vi "Process.vi"(8 "error in":errorcluster, 11 "instrument.PPMS2":refnum<class "instrument.PPMS2.lvclass">) -> (0 "error out":errorcluster, 3 "instrument.PPMS2 out":refnum<class "instrument.PPMS2.lvclass">)   [LabVIEW 2016, in "instrument.PPMS2.lvclass"]
doc: "---------------------------------------------------------------\nJKI State Machine Objects™\nhttp://jki.net/state-machine-objects/\nCopyright (C) 2005-2015, JKI <info@jki.net>\nALL RIGHTS RESERVED"
uses:
  instrument.PPMS2.lvclass
  C:/Program Files (x86)/National Instruments/LabVIEW 2016/vi.lib/JKI/JKI SMO/SMO/SMO.lvclass
  <vilib>/JKI/JKI SMO/SMO/Typedefs/Parent Call--Enum.ctl
  PPMS Global.vi
  C:/user/patrick/hg/levylab_inst_ppms2/lvsrc/QDInstrument_LabView/QDInstrument.dll
  QDInstrument_LabView/QDInstrument.dll
  <userlib>/LevyLab/Levylab Instruments DELETE ME SOMETIME/Instrument.lvclass
  <vilib>/JKI/JKI SMO/SMO/SMO.lvclass
panel:
  in  "Refresh Rate (Hz)":dbl=13.0
  out "Field Status":i32(ring)=1 items=["MagnetUnknown"=0, "StablePersistent"=1, "WarmingSwitch"=2, "CoolingSwitch"=3, "StableDriven"=4, "Iterating"=5, "Charging"=6, "Discharging"=7, "CurrentError"=8, "MagnetFailure"=15]
  in  "STOP":bool
  in  "Temp Approach":enum16{"FastSettle", "NoOvershoot"}(ring)
  in  "Low Helium Level Notify?":bool
  in  "Helium Notification Level":dbl=1.0
  out "Helium Level":dbl=86.7
  out "Position":dbl=90.002
  out "Field (Oe)":dbl=-0.00643419474363327 format="%_3g"
  out "Temperature(K)":dbl=305.0156 format="%#_5g"
  out "Temperature Status":T1(ring)=enum."Stable"
  in  "IP Address":string="130.49.180.72"
  # "PPMS2 Monitor Control"
  # "For instructions on how to use the JKI State Machine Objects, examples and video tutorials, visit:\nhttp://jki.net/state-machine-objects/\n\nJKI State Machine Objects™\nhttp://jki.net/state-machine-objects/\nCopyright (C) 2005-2015, JKI <info@jki.net>\nALL RIGHTS RESERVED"
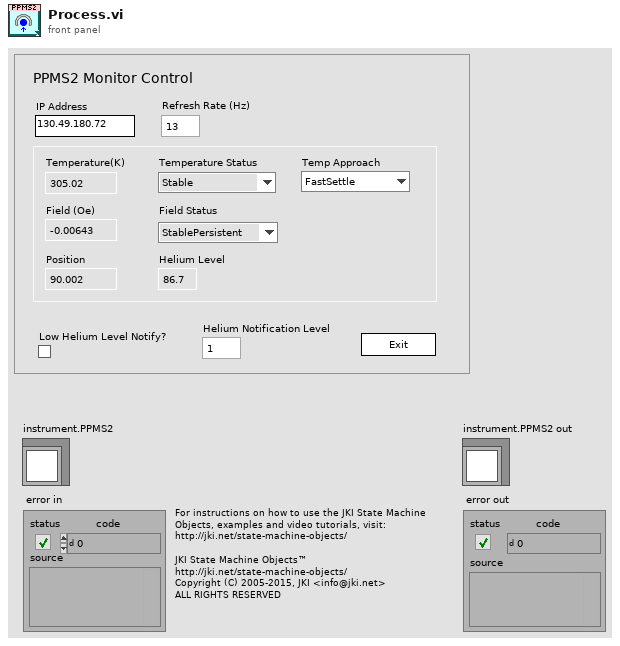
[diagram p1: front panel]
types:
  T1 = enum16{"TemperatureUnknown", "Stable", "Tracking", "Near", "Chasing", "Filling", "Standby", "Disabled", "ImpedanceNotFunction", "TempFailure"}
  T2 = typedef "SMO.lvclass/Parent Call--Enum.ctl" = enum16{"Allows parent to run", "Does not request parent to run"}
  T3 = enum32{"invalid app kind", "Development System", "Run Time System", "Student Edition", "Embedded LabVIEW", "Evaluation", "Custom"}
  T4 = enum32{"Invalid", "Standard", "Closed", "Hidden", "Minimized", "Maximized"}
  T5 = enum32{"Bad", "Idle", "Run top level", "Running"}
  T6 = enum16{"0", "1", "2", "3", "4", "5", "6", "7", "8", "9", "10", "11", "12", "13", "14"}
  T7 = cluster{"Core":cluster{"Current VI Reference":refnum<vi>, "Close Panel on Exit?":bool, "error":errorcluster}, "Self Reference":refnum<class "instrument.PPMS2.lvclass">, "to":i32, "Instrument Ref":refnum<k24>}
  T8 = cluster{"Current VI Reference":refnum<vi>, "Close Panel on Exit?":bool, "error":errorcluster}
  T9 = typedef "SMO.lvclass/Protected Events.ctl" = cluster{"StopProcesses":refnum<user-event>, "AbortProcesses":refnum<user-event>, "Config Changed":refnum<user-event>, "Dependency":refnum<user-event>}
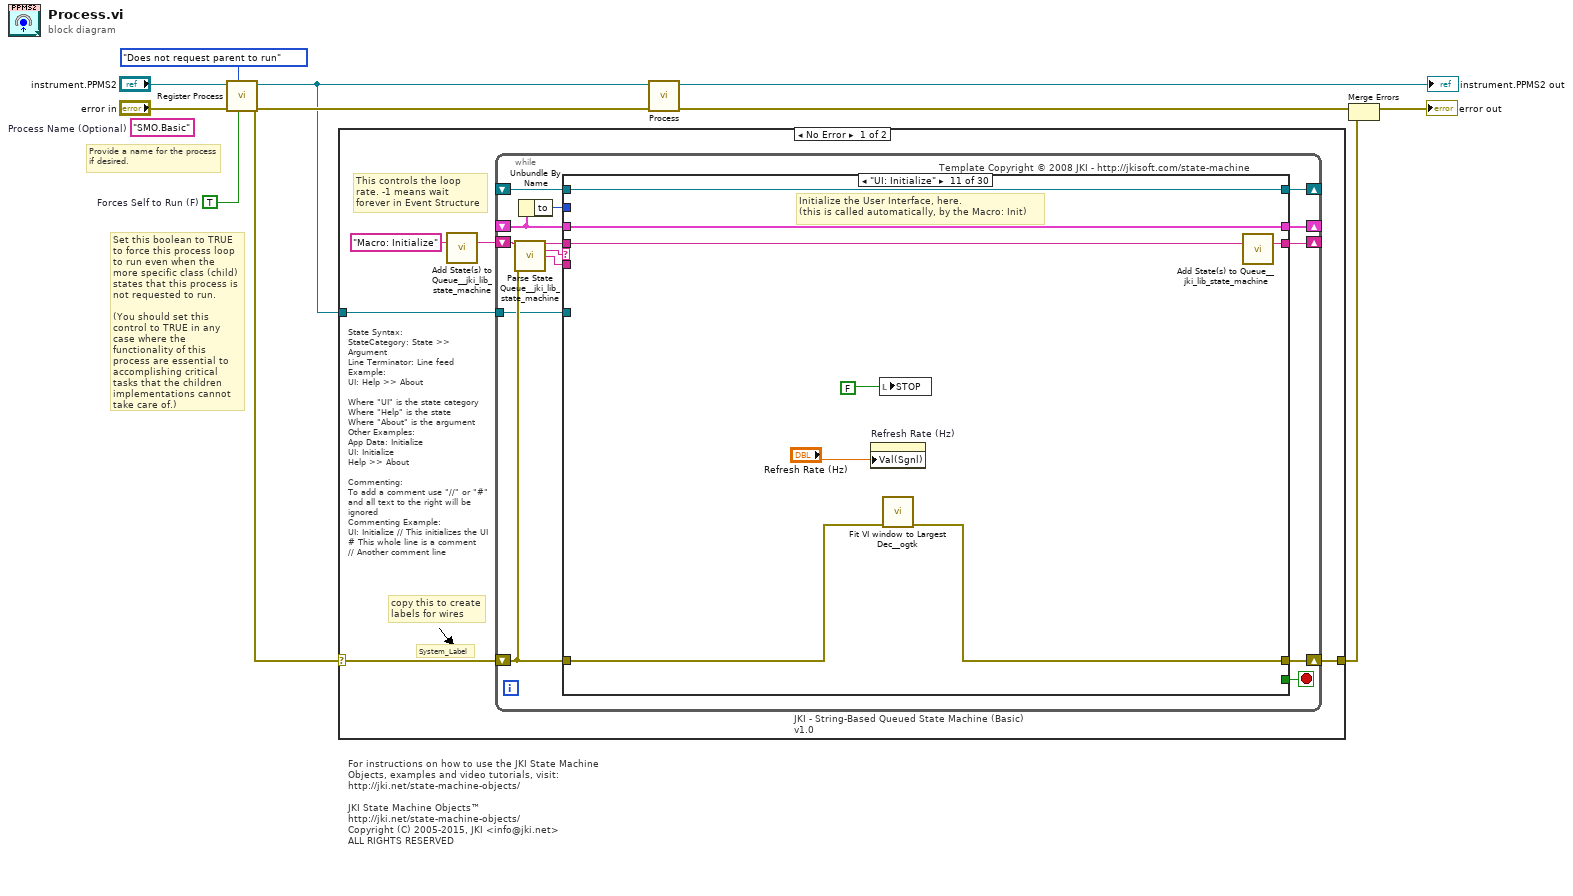
[diagram p0: block diagram]
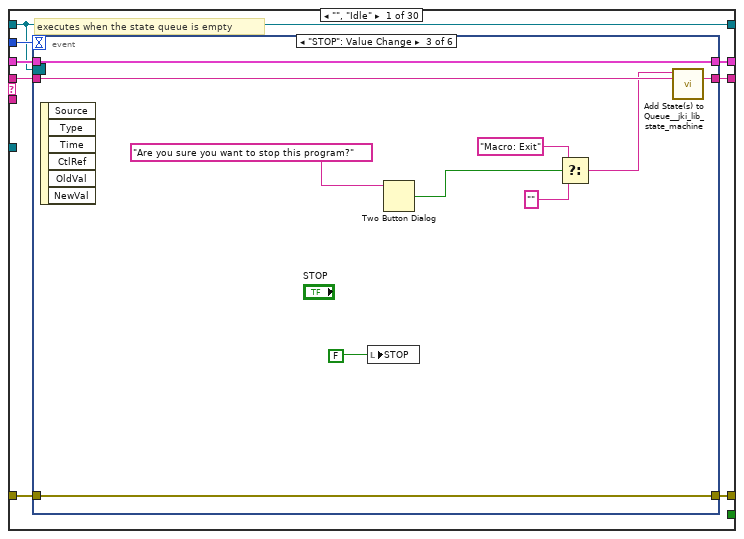
[diagram p2: hidden frame]
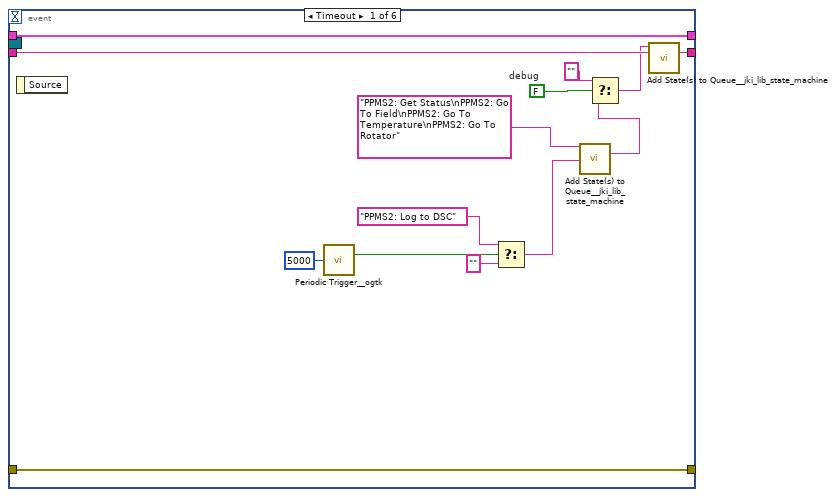
[diagram p3: hidden frame]
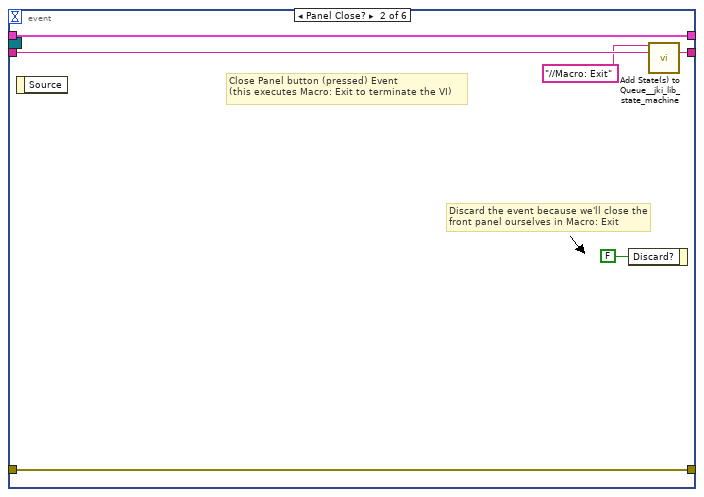
[diagram p4: hidden frame]
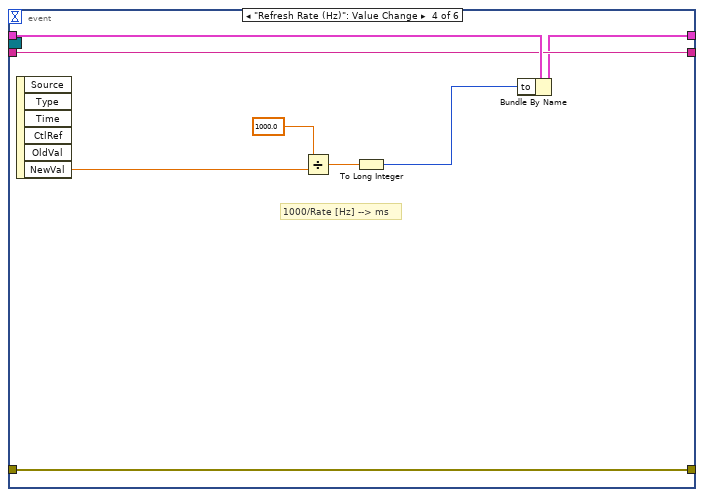
[diagram p5: hidden frame]
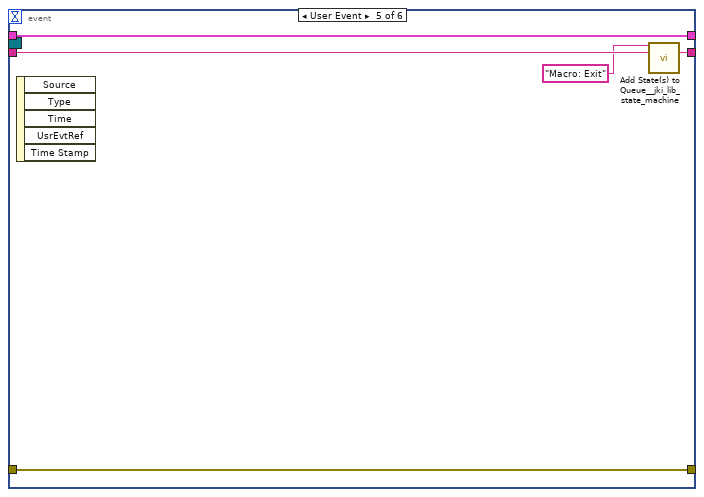
[diagram p6: hidden frame]
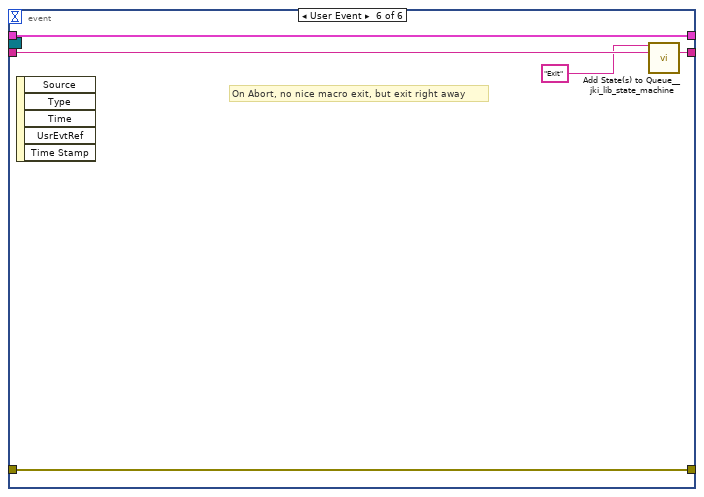
[diagram p7: hidden frame]
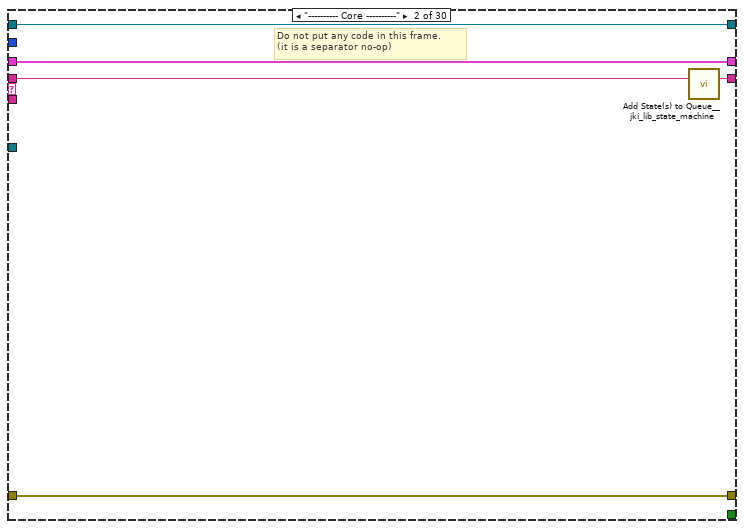
[diagram p8: hidden frame]
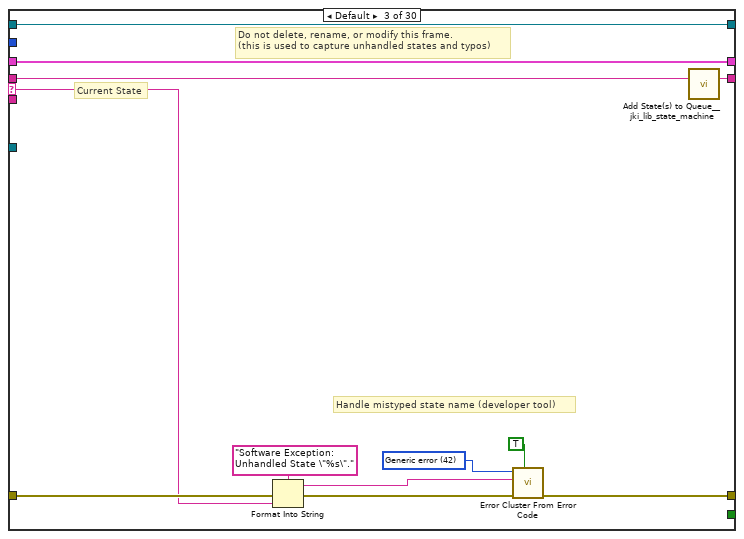
[diagram p9: hidden frame]
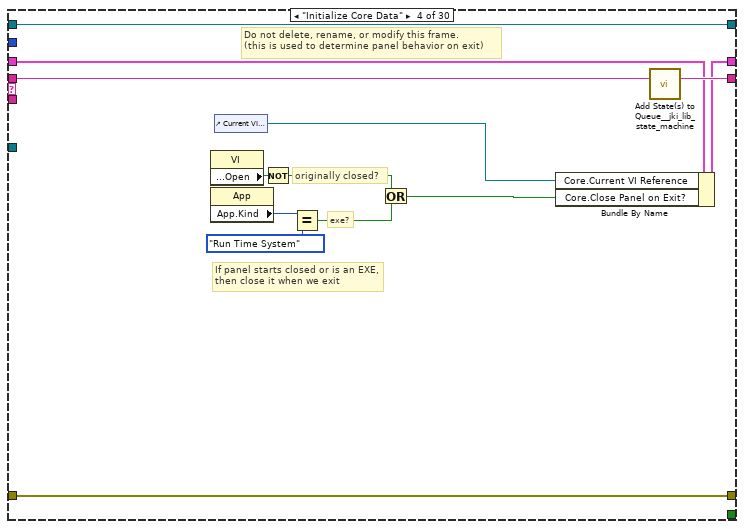
[diagram p10: hidden frame]
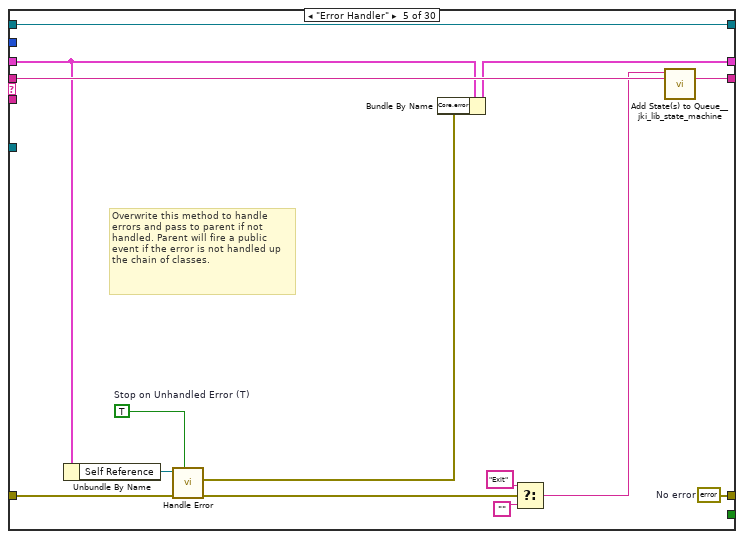
[diagram p11: hidden frame]
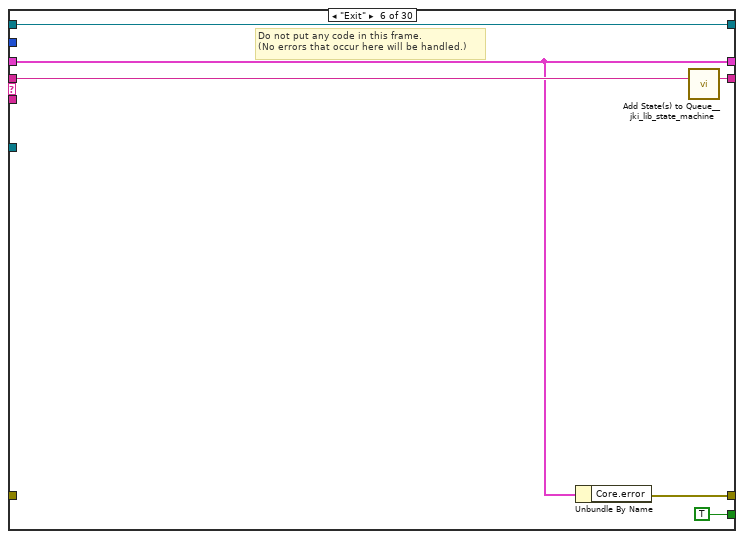
[diagram p12: hidden frame]
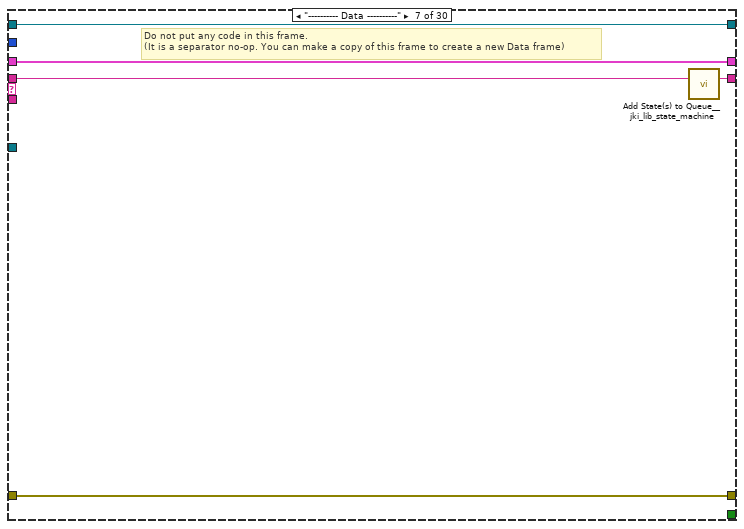
[diagram p13: hidden frame]
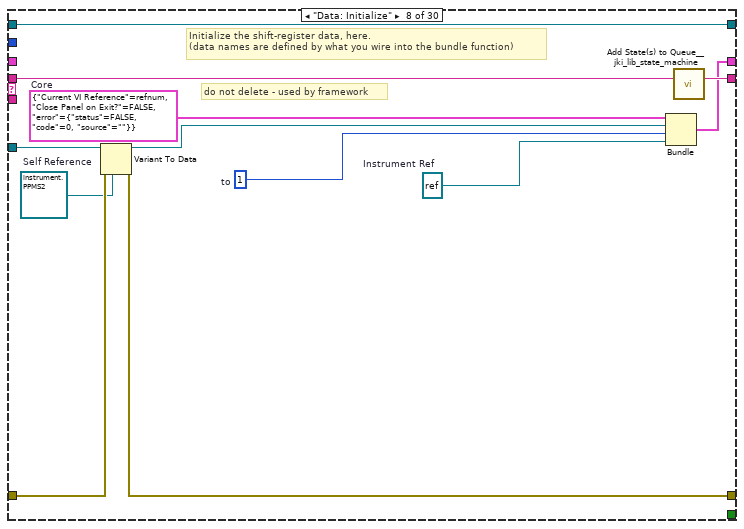
[diagram p14: hidden frame]
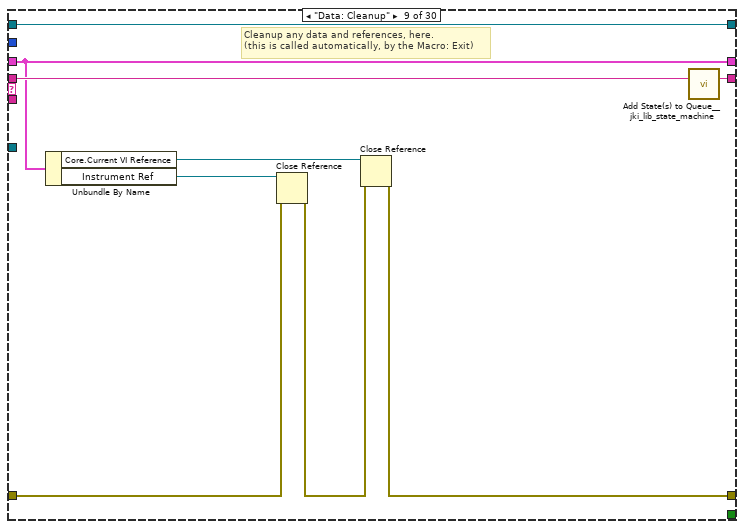
[diagram p15: hidden frame]
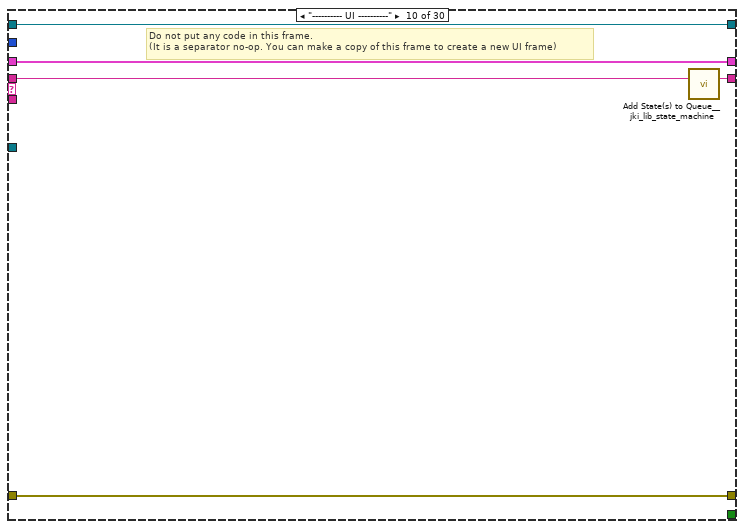
[diagram p16: hidden frame]
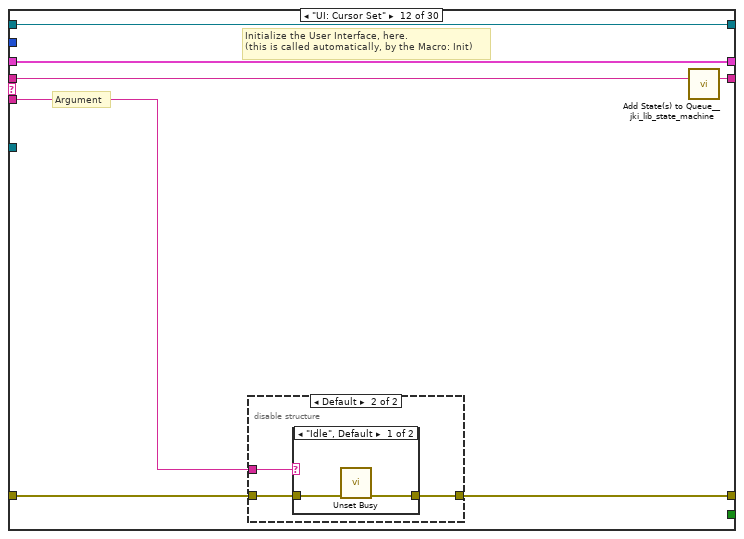
[diagram p17: hidden frame]
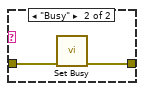
[diagram p19: hidden frame]
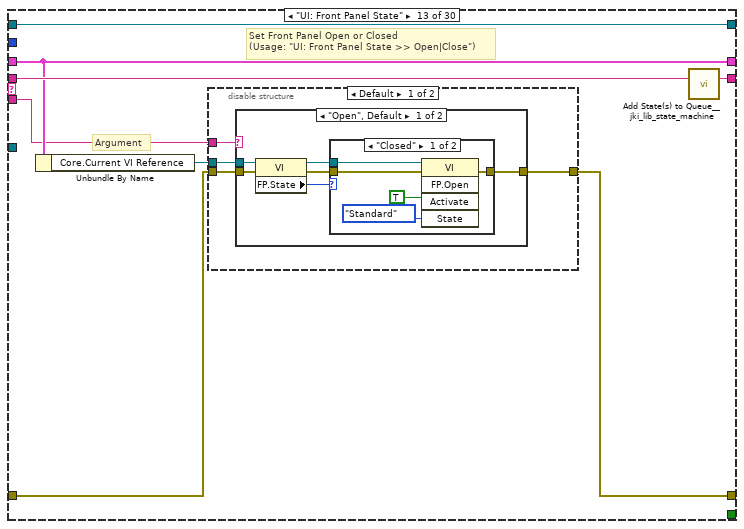
[diagram p20: hidden frame]
diagram:
  w1 = TRUE  # Forces Self to Run (F)
  (unwired) "SMO.Basic"  # Process Name (Optional)
  # "Provide a name for the process\nif desired."
  # "Set this boolean to TRUE to force this process loop to run even when the more specific class (child) states that this process is not requested to run.\n\n(You should set this control to TRUE in any case where the functionality of this process are essential to accomplishing critical tasks that the children implementations cannot take care of.)"
  # "For instructions on how to use the JKI State Machine Objects, examples and video tutorials, visit:\nhttp://jki.net/state-machine-objects/\n\nJKI State Machine Objects™\nhttp://jki.net/state-machine-objects/\nCopyright (C) 2005-2015, JKI <info@jki.net>\nALL RIGHTS RESERVED"
  n1 = call <vilib>:"Register Process.vi"("Forces Self to Run (F)"=w1, "Parent Call"=Parent_Call--Enum."Does not request parent to run", "error in (no error)"="error in", "SMO"="instrument.PPMS2") -> ("error out"=w7:errorcluster, "SMO out"=w6:refnum<class "instrument.PPMS2.lvclass">)  [unwired: 6 in]
  n2 = case shown="No Error" w7 {
    selector: w7 -> [w12 w466]
    tunnel: w6 -> [w13 _]
    tunnel: [w11 w466] -> w3
    frame No Error {
      # "State Syntax:\nStateCategory: State >> Argument\nLine Terminator: Line feed\nExample:\nUI: Help >> About\n\nWhere \"UI\" is the state category\nWhere \"Help\" is the state\nWhere \"About\" is the argument\nOther Examples:\nApp Data: Initialize\nUI: Initialize\nHelp >> About\n\nCommenting:\nTo add a comment use \"//\" or \"#\" and all text to the right will be ignored\nCommenting Example:\nUI: Initialize // This initializes the UI\n# This whole line is a comment\n// Another comment line"
      # "copy this to create labels for wires"
      # "This controls the loop rate. -1 means wait forever in Event Structure"
      # "System_Label"
      n3 = call <vilib>:"Add State(s) to Queue__jki_lib_state_machine.vi"("State(s) in (\"\")"="Macro: Initialize") -> ("States Out"=w15:string)  [unwired: 14 in]
      n4 = while "JKI - String-Based Queued State Machine (Basic) v1.0" {
        shift-right: [w22] -> _
        shift-left: _ -> [w17]
        shift-right: [w25] -> w11
        shift-left: w12 -> [w21]
        shift-right: [w24] -> _
        shift-left: w15 -> [w26]
        tunnel: w13 -> [w20]
        shift-right: [w19] -> _
        shift-left: _ -> [w18]
        stop <- w23 stop-if-true
        # "Template Copyright © 2008 JKI - http://jkisoft.com/state-machine"
        n5 = call <vilib>:"Parse State Queue__jki_lib_state_machine.vi"("State Queue"=w26, "Error In (no error)"=w21) -> ("Remaining States"=w28:string, "Current State"=w29:string, "Arguments"=w27:string)  [unwired: 11 in]
        n6 = Unbundle By Name(w17) -> ("to"=w16:i32)
        n7 = case shown="\"UI: Initialize\"" w29 {
          selector: w29 -> [_ _ w92 _ _ _ _ _ _ _ _ _ _ _ _ _ _ _ _ _ _ _ _ _ _ _ _ _ _ _]
          tunnel: w28 -> [w37 w90 w96 w115 w129 w135 w140 w152 w161 w166 w174 w181 w197 w229 w243 w257 w262 w269 w280 w285 w295 w301 w306 w317 w342 w363 w382 w400 w427 w465]
          tunnel: w27 -> [_ _ _ _ _ _ _ _ _ _ _ w175 w191 _ _ _ _ _ _ _ _ _ _ _ _ _ _ _ _ _]
          tunnel: w17 -> [w35 w87 w94 w106 w123 w131 w137 _ w157 w163 w172 w179 w193 w226 w239 w248 w259 w266 w277 w282 w293 w299 w304 w311 w339 w358 w377 w397 w425 w463]
          tunnel: [w34 w88 w98 w112 w124 w130 w138 w149 w158 w164 w169 w176 w194 w227 w241 w255 w260 w263 w271 w283 w288 w297 w302 w307 w337 w359 w378 w395 w423 w460] -> w25
          tunnel: w21 -> [w33 w88 w97 w112 w125 _ w138 w150 w154 w164 w170 w177 w195 w227 w241 w255 w260 w264 w272 w283 w289 w297 w302 w308 w338 w360 w379 w396 w423 w461]
          tunnel: [w36 w89 w95 w114 w128 w134 w139 w151 w160 w165 w173 w180 w196 w228 w242 w256 w261 w268 w279 w284 w294 w300 w305 w316 w341 w362 w381 w399 w426 w464] -> w24
          tunnel: [_ _ _ _ _ TRUE _ _ _ _ _ _ _ _ _ _ _ _ _ _ _ _ _ _ _ _ _ _ _ _] -> w23
          tunnel: [w32 w87 w94 w113 w122 w131 w137 w142 w157 w163 w172 w179 w193 w226 w239 w248 w259 w266 w277 w282 w293 w299 w304 w310 w339 w358 w377 w397 w425 w463] -> w22
          tunnel: w16 -> [w31 _ _ _ _ _ _ _ _ _ _ _ _ _ _ _ _ _ _ _ _ _ _ _ _ _ _ _ _ _]
          tunnel: w20 -> [_ _ _ _ _ _ _ w147 _ _ _ _ _ _ _ _ _ _ _ _ _ _ _ _ _ _ _ _ _ _]
          tunnel: [w30 w86 w91 w103 w127 w132 w136 w145 w156 w162 w171 w178 w190 w225 w240 w249 w258 w267 w278 w281 w292 w298 w303 w315 w340 w361 w380 w398 w424 w462] -> w19
          tunnel: w18 -> [w30 w86 w91 w103 w127 w132 w136 w145 w156 w162 w171 w178 w190 w225 w240 w249 w258 w267 w278 w281 _ w298 w303 w315 w340 w361 w380 w398 w424 w462]
          frame "", "Idle" {
            # "executes when the state queue is empty"
            n8 = event shown="[2] \"STOP\": Value Change" {
              selector: w30 -> [_ _ _ _ _ _]
              dyn-events: _ -> [_ _ _ _ _ _]
              timeout: w31 -> [_ _ _ _ _ _]
              tunnel: w37 -> [w51 w57 w67 w72 w80 w85]
              tunnel: [w50 w56 w66 w72 w79 w84] -> w36
              tunnel: w35 -> [w49 w54 w64 w73 w77 w82]
              tunnel: [w48 w55 w65 w68 w78 w83] -> w34
              tunnel: w33 -> [w48 w55 w65 w68 w78 w83]
              tunnel: [w49 w54 w64 w71 w77 w82] -> w32
              event Timeout {
                w40 = FALSE  # debug
                n9 = event-data() -> ()  [unwired: 1 in, 1 out]
                n10 = call <userlib>:"Periodic Trigger__ogtk.vi"("time (ms)"=u32 5000) -> ("Triggered"=w46:bool)  [unwired: 12 in, 2 out]
                n11 = Select(t="PPMS2: Log to DSC" ("State(s) in Front (\"\")"), s=w46, f="") -> (s? t:f=w42:string)
                n12 = call <vilib>:"Add State(s) to Queue__jki_lib_state_machine.vi"("State(s) in Front (\"\")"="PPMS2: Get Status\nPPMS2: Go To Field\nPPMS2: Go To Temperature\nPPMS2: Go To Rotator" ("State(s) in Front (\"\")"), "State(s) at Back (\"\")"=w42) -> ("States Out"=w39:string)  [unwired: 13 in]
                n13 = Select(t="" ("f"), s=w40, f=w39) -> (s? t:f=w38:string)
                n14 = call <vilib>:"Add State(s) to Queue__jki_lib_state_machine.vi"("State(s) in Front (\"\")"=w38, "State(s) in (\"\")"=w51) -> ("States Out"=w50:string)  [unwired: 13 in]
              }
              event Panel Close? {
                # "Discard the event because we'll close the front panel ourselves in Macro: Exit"
                # "Close Panel button (pressed) Event\n(this executes Macro: Exit to terminate the VI)"
                n15 = event-data() -> ()  [unwired: 1 in, 1 out]
                n16 = event-data("Discard?"=FALSE) -> ()  [unwired: 1 in, 1 out]
                n17 = call <vilib>:"Add State(s) to Queue__jki_lib_state_machine.vi"("State(s) in Front (\"\")"="//Macro: Exit", "State(s) in (\"\")"=w57) -> ("States Out"=w56:string)  [unwired: 13 in]
              }
              event "STOP": Value Change {
                n18 = event-data() -> ()  [unwired: 1 in, 6 out]
                n19 = local write "STOP"(FALSE ("STOP")) -> ()
                n20 = Two Button Dialog(message="Are you sure you want to stop this program?") -> (T button?=w63:bool)  [unwired: 2 in]
                n21 = Select(t="Macro: Exit", s=w63, f="") -> (s? t:f=w60:string)
                n22 = call <vilib>:"Add State(s) to Queue__jki_lib_state_machine.vi"("State(s) in Front (\"\")"=w60, "State(s) in (\"\")"=w67) -> ("States Out"=w66:string)  [unwired: 13 in]
              }
              event "Refresh Rate (Hz)": Value Change {
                # "1000/Rate [Hz] --> ms"
                n23 = event-data() -> ("NewVal"=w74:dbl)  [unwired: 1 in, 5 out]
                n24 = Divide(x=1000.0 ("milliseconds to wait"), y=w74) -> (x/y=w70:dbl)
                n25 = To Long Integer(number=w70) -> (32bit integer=w69:i32)
                n26 = Bundle By Name(cluster=w73, "to"=w69) -> (w71:T7)
              }
              event User Event {
                n27 = event-data() -> ()  [unwired: 1 in, 5 out]
                n28 = call <vilib>:"Add State(s) to Queue__jki_lib_state_machine.vi"("State(s) in Front (\"\")"="Macro: Exit", "State(s) in (\"\")"=w80) -> ("States Out"=w79:string)  [unwired: 13 in]
              }
              event User Event {
                # "On Abort, no nice macro exit, but exit right away"
                n29 = event-data() -> ()  [unwired: 1 in, 5 out]
                n30 = call <vilib>:"Add State(s) to Queue__jki_lib_state_machine.vi"("State(s) in Front (\"\")"="Exit", "State(s) in (\"\")"=w85) -> ("States Out"=w84:string)  [unwired: 13 in]
              }
            }
          }
          frame "---------- Core ----------" {
            # "Do not put any code in this frame.\n(it is a separator no-op)"
            n31 = call <vilib>:"Add State(s) to Queue__jki_lib_state_machine.vi"("State(s) in (\"\")"=w90) -> ("States Out"=w89:string)  [unwired: 14 in]
          }
          frame Default {
            w101 = 42 items=["No error", "Argument error", "Memory is full", "Out of zone", "End of file", "File already open", "Generic file I/O error", "File not found", "File permission error", "Disk is full", "Duplicate path", "Too many files open", "System feature not enabled", "Resource file not found", "Cannot add resource", "Resource not found", "Image not found", "Image memory error", "Pen does not exist", "Config type invalid", "Config token not found", "Config parse error", "Config memory error", "Bad external code format", "Bad external code offset", "External code not present", "Null window", "Destroy window error", "Null menu", "Print aborted", "Bad print record", "Print driver error", "Windows error during printing", "Memory error during printing", "Print dialog error", "Generic print error", "Invalid device refnum", "Device not found", "Device parameter error", "Device unit error", "Cannot open device", "Device call aborted", "Generic error", "Cancelled by user", "Object ID too low", "Object ID too high", "Object not in heap", "Unknown heap", "Unknown object (invalid DefProc)", "Unknown object (DefProc not in table)", "Message out of range", "Invalid (null) method", "Unknown message", "Manager call not supported", "Bad address", "Network operation in progress", "Network operation timed out", "Connection is busy", "Network attribute not supported", "Network error", "Address in use", "System out of memory", "Connection aborted", "Connection refused", "Not connected", "Already connected", "Connection closed", "Initialization error (interapplication manager)", "Bad occurrence", "Wait on unbound occurrence handler", "Occurrence queue overflow", "Datalog type conflict", "Unused", "Unrecognized type (interapplication manager)", "Memory corrupt", "Failed to make temporary DLL", "Old CIN version", "Drag socket not found", "Failed to load drop-object", "Failed to register OLE object", "Failed to release OLE object", "Format specifier type mismatch", "Unknown format specifier", "Too few format specifiers", "Too many format specifiers", "Scan failed", "Newer CIN version", "Error converting to variant", "Runtime menu error", "Password tampered", "Variant attribute not found", "Incompatible variant data type", "Event data is not available", "Event Store is not present", "Occurrence is not found", "Event Queue is not created", "Event info is not available", "Refnum passed is NULL", "Error retrieving Class GUID", "Error retrieving CoClass GUID", "Error retrieving TypeLib GUID.", "Bad built application magic bytes.", "Specific driver is different from the specific driver associated with the Logical Name.", "There is no session opened to the class driver.", "Max Error", "MAX - Error with config objects", "MAX - Error loading configuration", "MAX - Group not supported"]
            # "Current State"
            # "Do not delete, rename, or modify this frame.\n(this is used to capture unhandled states and typos)"
            # "Handle mistyped state name (developer tool)"
            n32 = Format Into String(format string="Software Exception: Unhandled State \"%s\"." ("message"), error in=w97, w92) -> (resulting string=w100:string, error out=w99:errorcluster)  [unwired: 1 in]
            n33 = call <vilib>:"Error Cluster From Error Code.vi"("show call chain? (False)"=TRUE, "error in (no error)"=w99, "error message (\"\")"=w100, "error code (0)"=w101) -> ("error out"=w98:errorcluster)  [unwired: 5 in]
            n34 = call <vilib>:"Add State(s) to Queue__jki_lib_state_machine.vi"("State(s) in (\"\")"=w96) -> ("States Out"=w95:string)  [unwired: 14 in]
          }
          frame "Initialize Core Data" {
            # "Do not delete, rename, or modify this frame.\n(this is used to determine panel behavior on exit)"
            # "originally closed?"
            # "exe?"
            # "If panel starts closed or is an EXE, then close it when we exit"
            n35 = property class="VI"() -> ("Front Panel.Open"=w111:bool)  [unwired: 2 in, 2 out]
            n36 = property class="App"() -> ("App.Kind"=w110:T3)  [unwired: 2 in, 2 out]
            n37 = control-ref of="Current VI Reference"() -> (w104:refnum<vi>)
            n38 = Not(x=w111) -> (.not. x?=w108:bool)
            n39 = Equal?(x=w110, y=T3."Run Time System" ("Application:Kind")) -> (x = y?=w107:bool)
            n40 = Or(x=w108, y=w107) -> (x .or. y?=w105:bool)
            n41 = Bundle By Name(cluster=w106, "Core.Current VI Reference"=w104, "Core.Close Panel on Exit?"=w105) -> (w113:T7)
            n42 = call <vilib>:"Add State(s) to Queue__jki_lib_state_machine.vi"("State(s) in (\"\")"=w115) -> ("States Out"=w114:string)  [unwired: 14 in]
          }
          frame "Error Handler" {
            w116 = TRUE  # Stop on Unhandled Error (T)
            w124 = errorcluster {"status"=FALSE, "code"=0, "source"=""}  # No error
            # "Overwrite this method to handle errors and pass to parent if not handled. Parent will fire a public event if the error is not handled up the chain of classes."
            n43 = Unbundle By Name(w123) -> ("Self Reference"=w126:refnum<class "instrument.PPMS2.lvclass">)
            n44 = call-dynamic "Handle Error.vi"("Stop on Unhandled Error (T)"=w116, "error in"=w125, "SMO"=w126) -> ("handling error"=w117:errorcluster, "Unhandled error"=w120:errorcluster)  [unwired: 6 in, 1 out]
            n45 = Bundle By Name(cluster=w123, "Core.error"=w120) -> (w122:T7)
            n46 = Select(t="Exit", s=w117, f="") -> (s? t:f=w121:string)
            n47 = call <vilib>:"Add State(s) to Queue__jki_lib_state_machine.vi"("State(s) in Front (\"\")"=w121, "State(s) in (\"\")"=w129) -> ("States Out"=w128:string)  [unwired: 13 in]
          }
          frame "Exit" {
            # "Do not put any code in this frame.\n(No errors that occur here will be handled.)"
            n48 = Unbundle By Name(w131) -> ("Core.error"=w130:errorcluster)
            n49 = call <vilib>:"Add State(s) to Queue__jki_lib_state_machine.vi"("State(s) in (\"\")"=w135) -> ("States Out"=w134:string)  [unwired: 14 in]
          }
          frame "---------- Data ----------" {
            # "Do not put any code in this frame.\n(It is a separator no-op. You can make a copy of this frame to create a new Data frame)"
            n50 = call <vilib>:"Add State(s) to Queue__jki_lib_state_machine.vi"("State(s) in (\"\")"=w140) -> ("States Out"=w139:string)  [unwired: 14 in]
          }
          frame "Data: Initialize" {
            w143 = refnum<k24> refnum  # Instrument Ref
            w144 = T8 {"Current VI Reference"=refnum, "Close Panel on Exit?"=FALSE, "error"={"status"=FALSE, "code"=0, "source"=""}}  # Core
            w148 = refnum<class "instrument.PPMS2.lvclass"> refnum  # Self Reference
            w141 = 1  # to
            # "do not delete - used by framework"
            # "Initialize the shift-register data, here.\n(data names are defined by what you wire into the bundle function)"
            n51 = Variant To Data(error in=w150, type=w148, Variant=w147) -> (data=w146:refnum<class "instrument.PPMS2.lvclass">, error out=w149:errorcluster)
            n52 = Bundle("Core"=w144, "Self Reference"=w146, "to"=w141, "Instrument Ref"=w143) -> (w142:T7)  [unwired: 1 in]
            n53 = call <vilib>:"Add State(s) to Queue__jki_lib_state_machine.vi"("State(s) in (\"\")"=w152) -> ("States Out"=w151:string)  [unwired: 14 in]
          }
          frame "Data: Cleanup" {
            # "Cleanup any data and references, here.\n(this is called automatically, by the Macro: Exit)"
            n54 = Unbundle By Name(w157) -> ("Core.Current VI Reference"=w159:refnum<vi>, "Instrument Ref"=w155:refnum<k24>)
            n55 = Close Reference(reference=w155, error in (no error)=w154) -> (error out=w153:errorcluster)
            n56 = Close Reference(reference=w159, error in (no error)=w153) -> (error out=w158:errorcluster)
            n57 = call <vilib>:"Add State(s) to Queue__jki_lib_state_machine.vi"("State(s) in (\"\")"=w161) -> ("States Out"=w160:string)  [unwired: 14 in]
          }
          frame "---------- UI ----------" {
            # "Do not put any code in this frame.\n(It is a separator no-op. You can make a copy of this frame to create a new UI frame)"
            n58 = call <vilib>:"Add State(s) to Queue__jki_lib_state_machine.vi"("State(s) in (\"\")"=w166) -> ("States Out"=w165:string)  [unwired: 14 in]
          }
          frame "UI: Initialize" {
            # "Initialize the User Interface, here.\n(this is called automatically, by the Macro: Init)"
            n59 = property on="Refresh Rate (Hz)" class="DigNum (strict)"("Val(Sgnl)"="Refresh Rate (Hz)") -> ()  [unwired: 2 in, 2 out]
            n60 = local write "STOP"(FALSE ("STOP")) -> ()
            n61 = call <userlib>:"Fit VI window to Largest Dec__ogtk.vi"("error in (no error)"=w170) -> ("error out"=w169:errorcluster)  [unwired: 5 in, 1 out]
            n62 = call <vilib>:"Add State(s) to Queue__jki_lib_state_machine.vi"("State(s) in (\"\")"=w174) -> ("States Out"=w173:string)  [unwired: 14 in]
          }
          frame "UI: Cursor Set" {
            # "Argument"
            # "Initialize the User Interface, here.\n(this is called automatically, by the Macro: Init)"
            n63 = disable-structure shown="Default" {
              disable-tunnel: w177 -> [w182 w185]
              disable-tunnel: [w182 w184] -> w176
              disable-tunnel: w175 -> [_ w183]
              frame condition #0 {
              }
              frame condition #1 (active) {
                n64 = case shown="\"Idle\", Default" w183 {
                  tunnel: w185 -> [w187 w189]
                  tunnel: [w186 w188] -> w184
                  frame "Idle", Default {
                    n65 = call <vilib>:"Unset Busy.vi"("error in (no error)"=w187) -> ("error out"=w186:errorcluster)  [unwired: 10 in]
                  }
                  frame "Busy" {
                    n66 = call <vilib>:"Set Busy.vi"("error in (no error)"=w189) -> ("error out"=w188:errorcluster)  [unwired: 9 in, 1 out]
                  }
                }
              }
            }
            n67 = call <vilib>:"Add State(s) to Queue__jki_lib_state_machine.vi"("State(s) in (\"\")"=w181) -> ("States Out"=w180:string)  [unwired: 14 in]
          }
          frame "UI: Front Panel State" {
            # "Argument"
            # "Set Front Panel Open or Closed\n(Usage: \"UI: Front Panel State >> Open|Close\")"
            n68 = Unbundle By Name(w193) -> ("Core.Current VI Reference"=w192:refnum<vi>)
            n69 = disable-structure shown="Default" {
              disable-tunnel: w195 -> [w201 w224]
              disable-tunnel: [w200 w224] -> w194
              disable-tunnel: w192 -> [w199 _]
              disable-tunnel: w191 -> [w198 _]
              frame condition #0 (active) {
                n70 = case shown="\"Open\", Default" w198 {
                  tunnel: w201 -> [w205 w218]
                  tunnel: [w207 w219] -> w200
                  tunnel: w199 -> [w206 w216]
                  frame "Open", Default {
                    n71 = property class="VI"(reference=w206, error in=w205) -> (reference out=w203:refnum<vi>, error out=w204:errorcluster, "FP.State"=w202:T4)
                    n72 = case shown="\"Closed\"" w202 {
                      tunnel: [w210 w213] -> w207
                      tunnel: w204 -> [w209 w213]
                      tunnel: w203 -> [w208 _]
                      frame "Closed" {
                        n73 = invoke class="VI" method="FP.Open"(reference=w208, error in=w209, "Activate"=TRUE, "State"=T4."Standard") -> (error out=w210:errorcluster)  [unwired: 1 in, 4 out]
                      }
                      frame Default {
                      }
                    }
                  }
                  frame "Close" {
                    n74 = property class="VI"(reference=w216, error in=w218) -> (reference out=w215:refnum<vi>, error out=w217:errorcluster, "FP.State"=w214:T4)
                    n75 = case shown="\"Invalid\", \"Closed\"" w214 {
                      tunnel: [w220 w223] -> w219
                      tunnel: w217 -> [w220 w222]
                      tunnel: w215 -> [_ w221]
                      frame "Invalid", "Closed" {
                      }
                      frame Default {
                        n76 = invoke class="VI" method="FP.Close"(reference=w221, error in=w222) -> (error out=w223:errorcluster)  [unwired: 1 in, 2 out]
                      }
                    }
                  }
                }
              }
              frame condition #1 {
              }
            }
            n77 = call <vilib>:"Add State(s) to Queue__jki_lib_state_machine.vi"("State(s) in (\"\")"=w197) -> ("States Out"=w196:string)  [unwired: 14 in]
          }
          frame "---------- Macro ----------" {
            # "Do not put any code in this frame.\n(It is a separator no-op. You can make a copy of this frame to create a new Macro frame)"
            n78 = call <vilib>:"Add State(s) to Queue__jki_lib_state_machine.vi"("State(s) in (\"\")"=w229) -> ("States Out"=w228:string)  [unwired: 14 in]
          }
          frame "Macro: Initialize" {
            w234 = "UI: Initialize\nUI: Front Panel State >> Open\nPPMS2: Initialize"  # UI: Initialize UI: Front Panel State >> Open PPMS2: Initialize
            w230 = "Process: Sync"
            # "Initialization Macro\n(This is called once, when the VI starts)"
            n79 = control-ref of="This VI"() -> (w232:refnum<vi>)
            n80 = property class="VI"(reference=w232) -> ("Exec.State"=w231:T5)  [unwired: 1 in, 2 out]
            n81 = Equal?(x=w231, y=T5."Run top level") -> (x = y?=w237:bool)
            n82 = Select(t=w230, s=w237, f="") -> ()  [unwired: 1 out]
            n83 = call <vilib>:"Add State(s) to Queue__jki_lib_state_machine.vi"("State(s) in Front (\"\")"="Data: Initialize\nInitialize Core Data\nEvents: Register", "State(s) in (\"\")"=w230, "State(s) at Back (\"\")"=w234) -> ("States Out"=w233:string)  [unwired: 12 in]
            n84 = call <vilib>:"Add State(s) to Queue__jki_lib_state_machine.vi"("State(s) in Front (\"\")"=w233, "State(s) in (\"\")"=w243) -> ("States Out"=w242:string)  [unwired: 13 in]
          }
          frame "Macro: Exit" {
            # "Exit Macro\n(This is called once, when the VI exits)"
            n85 = Unbundle By Name(w248) -> ("Core.Close Panel on Exit?"=w254:bool)
            n86 = Select(t="UI: Front Panel State >> Close", s=w254, f="") -> (s? t:f=w251:string)
            n87 = call <vilib>:"Add State(s) to Queue__jki_lib_state_machine.vi"("State(s) in Front (\"\")"="Data: Cleanup\nEvents: Unregister\nProcess: Self Terminate", "State(s) in (\"\")"="Process: Sync", "State(s) at Back (\"\")"="Exit") -> ("States Out"=w245:string)  [unwired: 12 in]
            n88 = call <vilib>:"Add State(s) to Queue__jki_lib_state_machine.vi"("State(s) in (\"\")"=w251, "State(s) at Back (\"\")"=w245) -> ("States Out"=w250:string)  [unwired: 13 in]
            n89 = call <vilib>:"Add State(s) to Queue__jki_lib_state_machine.vi"("State(s) in Front (\"\")"=w250, "State(s) in (\"\")"=w257) -> ("States Out"=w256:string)  [unwired: 13 in]
          }
          frame "---------- Process ----------" {
            # "Template Separator\n(You can make a copy of, or modify, this frame)"
            n90 = call <vilib>:"Add State(s) to Queue__jki_lib_state_machine.vi"("State(s) in (\"\")"=w262) -> ("States Out"=w261:string)  [unwired: 14 in]
          }
          frame "Process: Self Terminate" {
            n91 = Unbundle By Name(w266) -> ("Self Reference"=w265:refnum<class "instrument.PPMS2.lvclass">)
            n92 = call <vilib>:"SelfTerminate.vi"("error in (no error)"=w264, "SMO in"=w265) -> ("error out"=w263:errorcluster)  [unwired: 8 in, 1 out]
            n93 = call <vilib>:"Add State(s) to Queue__jki_lib_state_machine.vi"("State(s) in (\"\")"=w269) -> ("States Out"=w268:string)  [unwired: 14 in]
          }
          frame "Process: Sync" {
            n94 = Unbundle By Name(w277) -> ("Self Reference"=w273:refnum<class "instrument.PPMS2.lvclass">)
            n95 = call <vilib>:"WaitOnProcessSync.vi"("error in (no error)"=w272, "SMO"=w273) -> ("error out"=w271:errorcluster, "Don't run?"=w276:bool)  [unwired: 7 in, 1 out]
            n96 = Select(t="Data: Cleanup\nEvents: Unregister\nExit", s=w276, f="") -> (s? t:f=w270:string)
            n97 = call <vilib>:"Add State(s) to Queue__jki_lib_state_machine.vi"("State(s) in Front (\"\")"=w270, "State(s) in (\"\")"=w280) -> ("States Out"=w279:string)  [unwired: 13 in]
          }
          frame "---------- Events ----------" {
            # "Template Separator\n(You can make a copy of, or modify, this frame)"
            n98 = call <vilib>:"Add State(s) to Queue__jki_lib_state_machine.vi"("State(s) in (\"\")"=w285) -> ("States Out"=w284:string)  [unwired: 14 in]
          }
          frame "Events: Register" {
            # "Expand to add\nmore events"
            n99 = Unbundle By Name(w293) -> ("Self Reference"=w290:refnum<class "instrument.PPMS2.lvclass">)
            n100 = call <vilib>:"GetProtectedEvents.vi"("SMO"=w290) -> ("error out"=w286:errorcluster, "SMO Protected Events"=w291:T9)  [unwired: 8 in, 1 out]
            n101 = register-events(w291) -> (reference out=w292:refnum<event-registration>, error out=w287:errorcluster)  [unwired: 2 in]
            n102 = Merge Errors(w289, w287, w286) -> (w288:errorcluster)
            n103 = call <vilib>:"Add State(s) to Queue__jki_lib_state_machine.vi"("State(s) in (\"\")"=w295) -> ("States Out"=w294:string)  [unwired: 14 in]
          }
          frame "Events: Unregister" {
            n104 = Unregister For Events(event registration refnum=w298, error in=w297) -> (error out=w296:errorcluster)
            n105 = call <vilib>:"Clear Errors.vi"("error in (no error)"=w296) -> ()  [unwired: 5 in, 2 out]
            n106 = call <vilib>:"Add State(s) to Queue__jki_lib_state_machine.vi"("State(s) in (\"\")"=w301) -> ("States Out"=w300:string)  [unwired: 14 in]
          }
          frame "---------- PPMS2 ----------" {
            n107 = call <vilib>:"Add State(s) to Queue__jki_lib_state_machine.vi"("State(s) in (\"\")"=w306) -> ("States Out"=w305:string)  [unwired: 14 in]
          }
          frame "PPMS2: Initialize" {
            w312 = 0 items=["PPMS", "VersaLab", "DynaCool", "SVSM"] ("Instrument\nType")
            n108 = call "OpenQDInstrument.vi"("Remote"=TRUE, "IP Address"="IP Address", "Instrument Type"=w312, "error in (no error)"=w308) -> ("error out"=w307:errorcluster, "Instrument Ref"=w314:refnum<k24>)  [unwired: 4 in]
            n109 = Bundle By Name(cluster=w311, "Instrument Ref"=w314) -> (w310:T7)
            n110 = call <vilib>:"Add State(s) to Queue__jki_lib_state_machine.vi"("State(s) in (\"\")"=w317) -> ("States Out"=w316:string)  [unwired: 14 in]
          }
          frame "PPMS2: Get Status" {
            n111 = Unbundle By Name(w339) -> ("Instrument Ref"=w335:refnum<k24>)
            n112 = call "GetTemperature.vi"("error in (no error)"=w338, "Instrument Ref In"=w335) -> ("Temperature\nStatus"=→"Temperature Status":i32, "Temperature"=w322:dbl, "error out"=w334:errorcluster, "Instrument Ref Out"=w333:refnum<k24>)  [unwired: 3 in, 1 out]
            "Temperature(K)" <- w322
            n113 = call "GetField.vi"("error in (no error)"=w334, "Instrument Ref In"=w333) -> ("Field\nStatus"=→"Field Status":i32, "Field"=w321:dbl, "error out"=w330:errorcluster, "Instrument Ref Out"=w331:refnum<k24>)  [unwired: 3 in, 1 out]
            "Field (Oe)" <- w321
            n114 = global write "PPMS Global.vi" "Temperature (K)"(w322) -> ()
            n115 = global write "PPMS Global.vi" "Field (Oe)"(w321) -> ()
            n116 = call "GetPPMSItem.vi"("Channel"=3, "error in (no error)"=w330, "Instrument Ref In"=w331) -> ("Result"=w318:dbl, "error out"=w326:errorcluster, "Instrument Ref Out"=w327:refnum<k24>)  [unwired: 1 in, 1 out]
            "Position" <- w318
            n117 = global write "PPMS Global.vi" "Position (Degree)"(w318) -> ()
            n118 = call "SendPPMSCommand.vi"("PpmsCommand"="LEVEL?", "error in (no error)"=w326, "Instrument Ref In"=w327) -> ("PpmsReply"=w336:string, "error out"=w337:errorcluster)  [unwired: 4 in, 3 out]
            n119 = Match Pattern(string=w336, regular expression=",") -> (before substring=w324:string)  [unwired: 1 in, 3 out]
            n120 = global write "PPMS Global.vi" "Helium Level String"(w324) -> ()
            n121 = Scan Value(string=w324, format string="%g") -> (value=w319:dbl)  [unwired: 1 in, 1 out]
            "Helium Level" <- w319
            n122 = global write "PPMS Global.vi" "Helium Level"(w319) -> ()
            n123 = call <vilib>:"Add State(s) to Queue__jki_lib_state_machine.vi"("State(s) in (\"\")"=w342) -> ("States Out"=w341:string)  [unwired: 14 in]
          }
          frame "PPMS2: Go To Field" {
            n124 = Unbundle By Name(w358) -> ("Instrument Ref"=w344:refnum<k24>)
            n125 = global read "PPMS Global.vi" "Target Field"() -> (w353:dbl)
            n126 = global read "PPMS Global.vi" "Helium Level"() -> (w347:dbl)
            n127 = global read "PPMS Global.vi" "Set Field?"() -> (w348:bool)
            n128 = global read "PPMS Global.vi" "Field (Oe)"() -> (w357:dbl)
            n129 = Absolute Value(x=w353) -> (abs(x)=w352:dbl)
            n130 = Greater?(x=w347, y=70) -> (0:w345:bool)
            n131 = Subtract(x=w353, y=w357) -> (x-y=w356:dbl)
            n132 = Less Or Equal?(x=w352, y=70000.0) -> (x <= y?=w349:bool)
            n133 = Absolute Value(x=w356) -> (abs(x)=w355:dbl)
            n134 = Greater?(x=w355, y=10.0) -> (0:w350:bool)
            n135 = Compound Arithmetic op=AND(w345, w349, w350, w348) -> (w343:bool)
            n136 = case shown="True" w343 {
              tunnel: w344 -> [w365 w372]
              tunnel: w360 -> [w364 w371]
              tunnel: [w365 w368] -> _
              tunnel: [w364 w367] -> w359
              frame False {
              }
              frame True {
                w373 = 0 items=["Linear", "NoOvershoot", "Oscillate"] ("Approach")
                w374 = 0 items=["Persistent", "Driven"] ("Mode")
                n137 = global read "PPMS Global.vi" "Target Field"() -> (w370:dbl)
                n138 = global read "PPMS Global.vi" "Rate (Oe/s)"() -> (w369:dbl)
                n139 = global write "PPMS Global.vi" "Set Field?"(FALSE ("Set Field?")) -> ()
                n140 = call "SetField.vi"("Mode"=w374, "Approach"=w373, "Rate"=w369, "Field"=w370, "error in (no error)"=w371, "Instrument Ref In"=w372) -> ("error out"=w367:errorcluster, "Instrument Ref Out"=w368:refnum<k24>)  [unwired: 1 in, 1 out]
              }
            }
            n141 = call <vilib>:"Add State(s) to Queue__jki_lib_state_machine.vi"("State(s) in (\"\")"=w363) -> ("States Out"=w362:string)  [unwired: 14 in]
          }
          frame "PPMS2: Go To Temperature" {
            n142 = Unbundle By Name(w377) -> ("Instrument Ref"=w376:refnum<k24>)
            n143 = global read "PPMS Global.vi" "Set Temp?"() -> (w375:bool)
            n144 = case shown="True" w375 {
              tunnel: w376 -> [w384 w392]
              tunnel: w379 -> [w383 w391]
              tunnel: [w384 w388] -> _
              tunnel: [w383 w387] -> w378
              frame False {
              }
              frame True {
                n145 = global read "PPMS Global.vi" "Rate (K/min)"() -> (w389:dbl)
                n146 = global read "PPMS Global.vi" "Target Temp"() -> (w390:dbl)
                n147 = global write "PPMS Global.vi" "Set Temp?"(FALSE ("Set Field?")) -> ()
                n148 = call "SetTemperature.vi"("Approach"="Temp Approach", "Rate"=w389, "Temperature"=w390, "error in (no error)"=w391, "Instrument Ref In"=w392) -> ("error out"=w387:errorcluster, "Instrument Ref Out"=w388:refnum<k24>)  [unwired: 2 in, 1 out]
              }
            }
            n149 = call <vilib>:"Add State(s) to Queue__jki_lib_state_machine.vi"("State(s) in (\"\")"=w382) -> ("States Out"=w381:string)  [unwired: 14 in]
          }
          frame "PPMS2: Go To Rotator" {
            n150 = Unbundle By Name(w397) -> ("Instrument Ref"=w394:refnum<k24>)
            n151 = global read "PPMS Global.vi" "Set Position?"() -> (w393:bool)
            n152 = case shown="True" w393 {
              tunnel: w394 -> [w402 w407]
              tunnel: w396 -> [w401 w406]
              tunnel: [w402 w405] -> _
              tunnel: [w401 w404] -> w395
              frame False {
              }
              frame True {
                w412 = u16 0 items=["Move to position", "Move to limit", "Redefine current position", ""] ("Mode")
                n153 = global read "PPMS Global.vi" "Target Position"() -> (w408:dbl)
                n154 = Number To Decimal String(number=w408) -> (decimal integer string=w410:string)  [unwired: 1 in]
                n155 = Number To Decimal String(number=w412) -> (decimal integer string=w413:string)  [unwired: 1 in]
                n156 = Number To Decimal String(number=T6."0" ("Slow down code\ndefault = 0")) -> (decimal integer string=w416:string)  [unwired: 1 in]
                n157 = Concatenate Strings("MOVE " ("string"), w410, " " ("string"), w413, " " ("string"), w416) -> (w417:string)
                n158 = global write "PPMS Global.vi" "Set Position?"(FALSE ("Set Field?")) -> ()
                n159 = call "SendPPMSCommand.vi"("PpmsCommand"=w417, "error in (no error)"=w406, "Instrument Ref In"=w407) -> ("error out"=w404:errorcluster, "Instrument Ref Out"=w405:refnum<k24>)  [unwired: 4 in, 3 out]
              }
            }
            n160 = call <vilib>:"Add State(s) to Queue__jki_lib_state_machine.vi"("State(s) in (\"\")"=w400) -> ("States Out"=w399:string)  [unwired: 14 in]
          }
          frame "PPMS2: Low Helium" {
            # "Send low helium level notification"
            n161 = global read "PPMS Global.vi" "Helium Level"() -> (w422:dbl)
            n162 = Less?(x=w422, y="Helium Notification Level") -> (x < y?=w420:bool)
            n163 = And(x=w420, y="Low Helium Level Notify?") -> (x .and. y?=w421:bool)
            n164 = case shown="True" w421 {
              frame False {
              }
              frame True {
                n165 = local write "Low Helium Level Notify?"(FALSE ("Low Helium Level Notify?")) -> ()
              }
            }
            n166 = call <vilib>:"Add State(s) to Queue__jki_lib_state_machine.vi"("State(s) in (\"\")"=w427) -> ("States Out"=w426:string)  [unwired: 14 in]
          }
          frame "PPMS2: Log To DSC" {
            n167 = global read "PPMS Global.vi" "Position (Degree)"() -> (w459:dbl)
            n168 = shared-variable-open(refnum<k21> "ni.var.psp://housesoftheholy/PPMS 2/PPMS 2 Position" ("shared variable refnum in"), w461, 0.0) -> (w455:refnum<k21>, w439:errorcluster)  [unwired: 1 in]
            n169 = shared-variable-write(w455, w439, w459) -> (w456:refnum<k21>, w438:errorcluster)
            n170 = Close Variable Connection(8:w438, 11:w456) -> (0:w437:errorcluster)
            n171 = global read "PPMS Global.vi" "Temperature (K)"() -> (w449:dbl)
            n172 = shared-variable-open(refnum<k21> "ni.var.psp://housesoftheholy/PPMS 2/PPMS 2 Temperature" ("shared variable refnum in"), w437, 0.0) -> (w445:refnum<k21>, w436:errorcluster)  [unwired: 1 in]
            n173 = global read "PPMS Global.vi" "Field (Oe)"() -> (w441:dbl)
            n174 = shared-variable-write(w445, w436, w449) -> (w446:refnum<k21>, w435:errorcluster)
            n175 = Close Variable Connection(8:w435, 11:w446) -> (0:w434:errorcluster)
            n176 = shared-variable-open(refnum<k21> "ni.var.psp://housesoftheholy/PPMS 2/PPMS 2 Magnetic Field" ("shared variable refnum in"), w434, 0.0) -> (w442:refnum<k21>, w433:errorcluster)  [unwired: 1 in]
            n177 = shared-variable-write(w442, w433, w441) -> (w443:refnum<k21>, w432:errorcluster)
            n178 = global read "PPMS Global.vi" "Helium Level"() -> (w454:dbl)
            n179 = Close Variable Connection(8:w432, 11:w443) -> (0:w431:errorcluster)
            n180 = shared-variable-open(refnum<k21> "ni.var.psp://housesoftheholy/PPMS 2/PPMS 2 Helium Level" ("shared variable refnum in"), w431, 0.0) -> (w450:refnum<k21>, w430:errorcluster)  [unwired: 1 in]
            n181 = shared-variable-write(w450, w430, w454) -> (w451:refnum<k21>, w429:errorcluster)
            n182 = Close Variable Connection(8:w429, 11:w451) -> (0:w460:errorcluster)
            n183 = call <vilib>:"Add State(s) to Queue__jki_lib_state_machine.vi"("State(s) in (\"\")"=w465) -> ("States Out"=w464:string)  [unwired: 14 in]
          }
        }
      }
    }
    frame Error {
    }
  }
  n184 = call-parent "Process.vi"("error in"=w7, "Instrument"=w6) -> ("error out"=w4:errorcluster, "Instrument out"=→"instrument.PPMS2 out":refnum<class "instrument.PPMS2.lvclass">)  [unwired: 8 in]
  n185 = Merge Errors(w4, w3) -> (→"error out":errorcluster)
